vi "Initialize.vi"(0 "VISA resource name":refnum<visa-resource-name>, 1 "Reset to Default (False)":bool, 5 "ID Query (True)":bool=TRUE, 7 "Reset (True)":bool=TRUE, 11 "error in (no error)":errorcluster, 12 "Baud Rate (2: 9600)":i32(ring)=2 items=["300", "1200", "9600"]) -> (4 "VISA resource name out":refnum<visa-resource-name>, 15 "error out":errorcluster)   [LabVIEW 2019, in "Lake Shore Cryotronics 370.lvlib"]
doc: "This VI passes the addressing information in the instrument decriptor to the Instr Open VI and returns the instrument ID. You can optionally reset the instrument by setting the front panel reset control. You must run this VI before using any of the instrument driver VIs for this instrument.\n\nNOTE: If you do not want the instrument reset to its default setup state you MUST set the Reset Defaults control to FALSE."
uses:
  Lake Shore Cryotronics 370.lvlib
panel:
  # "(c) 2001- 2009 National Instruments.  ALL RIGHTS RESERVED."
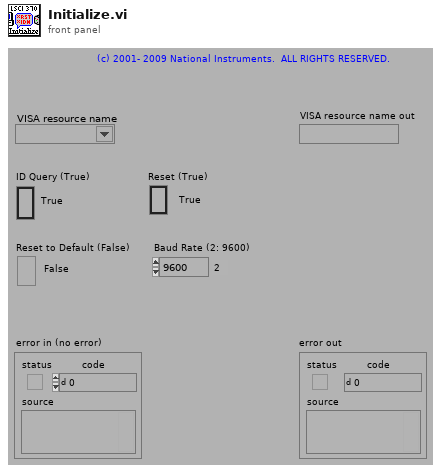
[diagram p1: front panel]
types:
  T1 = cluster{"Status":bool, "Code":i32, "Source (VI Name)":string}
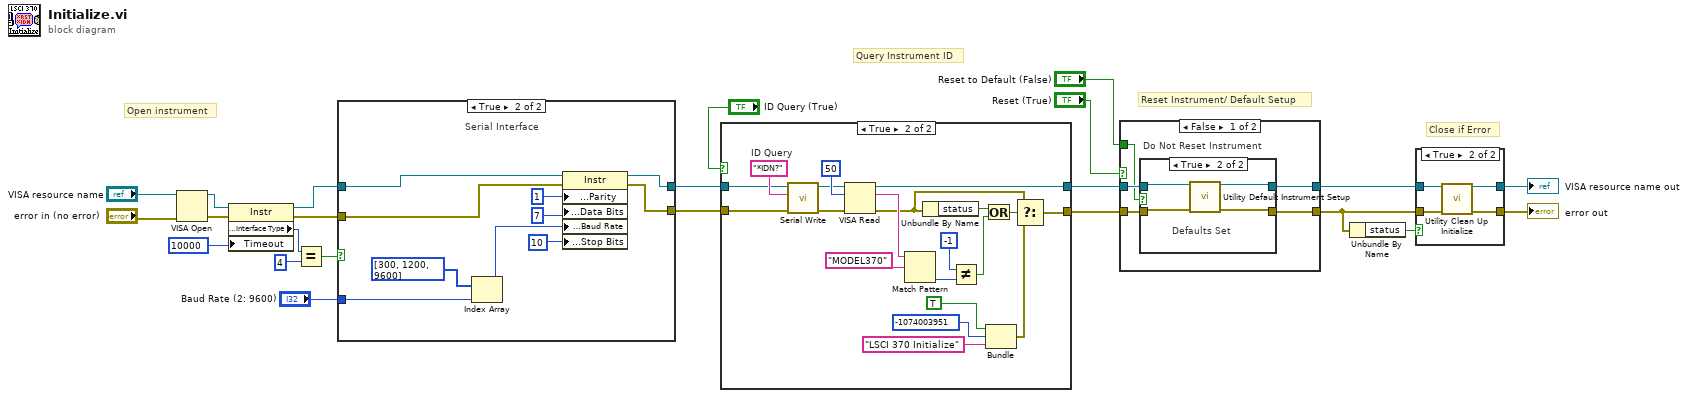
[diagram p0: block diagram]
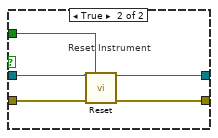
[diagram p5: hidden frame]
diagram:
  # "Close if Error"
  # "Reset Instrument/ Default Setup"
  # "Query Instrument ID"
  # "Open instrument"
  n1 = VISA Open(error in (no error)="error in (no error)", VISA resource name="VISA resource name") -> (VISA resource name=w5:refnum<visa-resource-name>, error out=w4:errorcluster)  [unwired: 3 in]
  n2 = property class="Instr"(reference=w5, error in=w4, "Timeout"=u32 10000 ("Tmo Value")) -> (reference out=w10:refnum<visa-resource-name>, error out=w11:errorcluster, "Interface Information:Interface Type"=w13:u16)
  n3 = Equal?(x=w13, y=4) -> (x = y?=w12:bool)
  n4 = case shown="True" w12 {
    tunnel: w11 -> [w25 w31]
    tunnel: [w25 w28] -> w8
    tunnel: w10 -> [w24 w30]
    tunnel: [w24 w29] -> w9
    tunnel: "Baud Rate (2: 9600)" -> [_ w26]
    frame False {
      # "GPIB Interface"
    }
    frame True {
      # "Serial Interface"
      n5 = Index Array(array=u32[] [300, 1200, 9600], index=w26) -> (element=w33:u32)
      n6 = property class="Instr"(reference=w30, error in=w31, "Serial Settings:Parity"=1, "Serial Settings:Data Bits"=u16 7, "Serial Settings:Baud Rate"=w33, "Serial Settings:Stop Bits"=10) -> (reference out=w29:refnum<visa-resource-name>, error out=w28:errorcluster)
    }
  }
  n7 = case shown="True" "ID Query (True)" {
    tunnel: [w36 w57] -> w22
    tunnel: [w37 w56] -> w23
    tunnel: w9 -> [w37 w39]
    tunnel: w8 -> [w36 w38]
    frame False {
    }
    frame True {
      w40 = "*IDN?"  # ID Query
      n8 = call "Serial Write.vi"("error in (no error)"=w38, "Write Buffer (\"\")"=w40, "VISA resource name"=w39) -> ("error out"=w42:errorcluster, "VISA resource name out"=w41:refnum<visa-resource-name>)  [unwired: 6 in, 1 out]
      n9 = VISA Read(VISA resource name=w41, byte count=u32 50, error in (no error)=w42) -> (VISA resource name out=w56:refnum<visa-resource-name>, read buffer=w53:string, error out=w52:errorcluster)  [unwired: 1 out]
      n10 = Match Pattern(string=w53, regular expression="MODEL370") -> (offset past match=w47:i32)  [unwired: 1 in, 3 out]
      n11 = Unbundle By Name(w52) -> ("status"=w50:bool)
      n12 = Not Equal?(x=-1, y=w47) -> (x != y?=w54:bool)
      n13 = Or(x=w50, y=w54) -> (x .or. y?=w51:bool)
      n14 = Bundle("Status"=TRUE, "Code"=-1074003951, "Source (VI Name)"="LSCI 370 Initialize") -> (w45:T1)  [unwired: 1 in]
      n15 = Select(t=w52, s=w51, f=w45) -> (s? t:f=w57:T1)
    }
  }
  n16 = case shown="False" "Reset (True)" {
    tunnel: w22 -> [w61 w72]
    tunnel: [w60 w71] -> w18
    tunnel: w23 -> [w62 w73]
    tunnel: [w59 w70] -> w17
    tunnel: "Reset to Default (False)" -> [w58 w69]
    frame False {
      # "Do Not Reset Instrument"
      n17 = case shown="True" w58 {
        tunnel: w62 -> [w64 w68]
        tunnel: w61 -> [w63 w67]
        tunnel: [w63 w66] -> w60
        tunnel: [w64 w65] -> w59
        frame False {
          # "No Defaults Set"
        }
        frame True {
          # "Defaults Set"
          n18 = call "Utility Default Instrument Setup.vi"("VISA resource name"=w68, "error in (no error)"=w67) -> ("VISA resource name out"=w65:refnum<visa-resource-name>, "error out"=w66:errorcluster)  [unwired: 12 in]
        }
      }
    }
    frame True {
      # "Reset Instrument"
      n19 = call "Reset.vi"("VISA resource name"=w73, "Reset to Default (False)"=w69, "error in (no error)"=w72) -> ("VISA resource name out"=w70:refnum<visa-resource-name>, "error out"=w71:errorcluster)  [unwired: 11 in]
    }
  }
  n20 = Unbundle By Name(w18) -> ("status"=w19:bool)
  n21 = case shown="True" w19 {
    tunnel: w17 -> [w75 w79]
    tunnel: w18 -> [w74 w78]
    tunnel: [w75 w76] -> w16
    tunnel: [w74 w77] -> w15
    frame False {
    }
    frame True {
      n22 = call "Utility Clean Up Initialize.vi"("VISA session"=w79, "error in (no error)"=w78) -> ("dup VISA session"=w76:refnum<visa-resource-name>, "error out"=w77:errorcluster)  [unwired: 12 in]
    }
  }
  "VISA resource name out" <- w16
  "error out" <- w15
